vi "lab15_3-21_main.vi"() -> ()   [LabVIEW 2012]
uses:
  <vilib>/DAQmx/write.llb/DAQmx Write (Digital U8 1Chan 1Samp).vi
  <vilib>/DAQmx/create/channels.llb/DAQmx Create Channel (DO-Digital Output).vi
  <vilib>/DAQmx/miscellaneous.llb/DAQmx Fill In Error Info.vi
panel:
  out "out":u8 format="%08b"
  in  "Half-stepping":bool
  in  "Digital Port":tag
  in  "Number of steps\n(0 for run mode)":i32(knob) min=0 max=1000 scale=0.0..50.0
  in  "Stop Movement":bool
  in  "Move Right":bool
  in  "Move Left":bool
  in  "Terminate Program":bool
  in  "Speed":u8(knob)=1 max=7 step=1 scale=0.0..7.0
  # "Channel Configuration"
  # "Motor Operation"
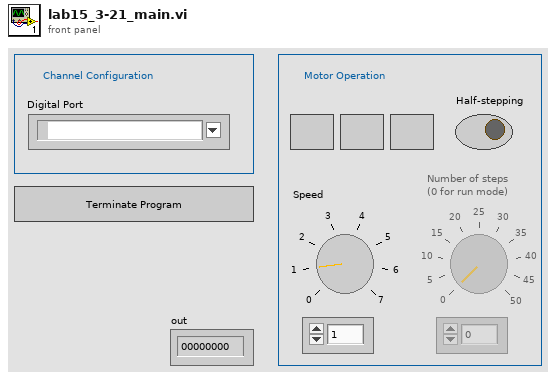
[diagram p1: front panel]
types:
  T1 = enum8{"Enabled", "Disabled", "Disabled and Grayed Out"}
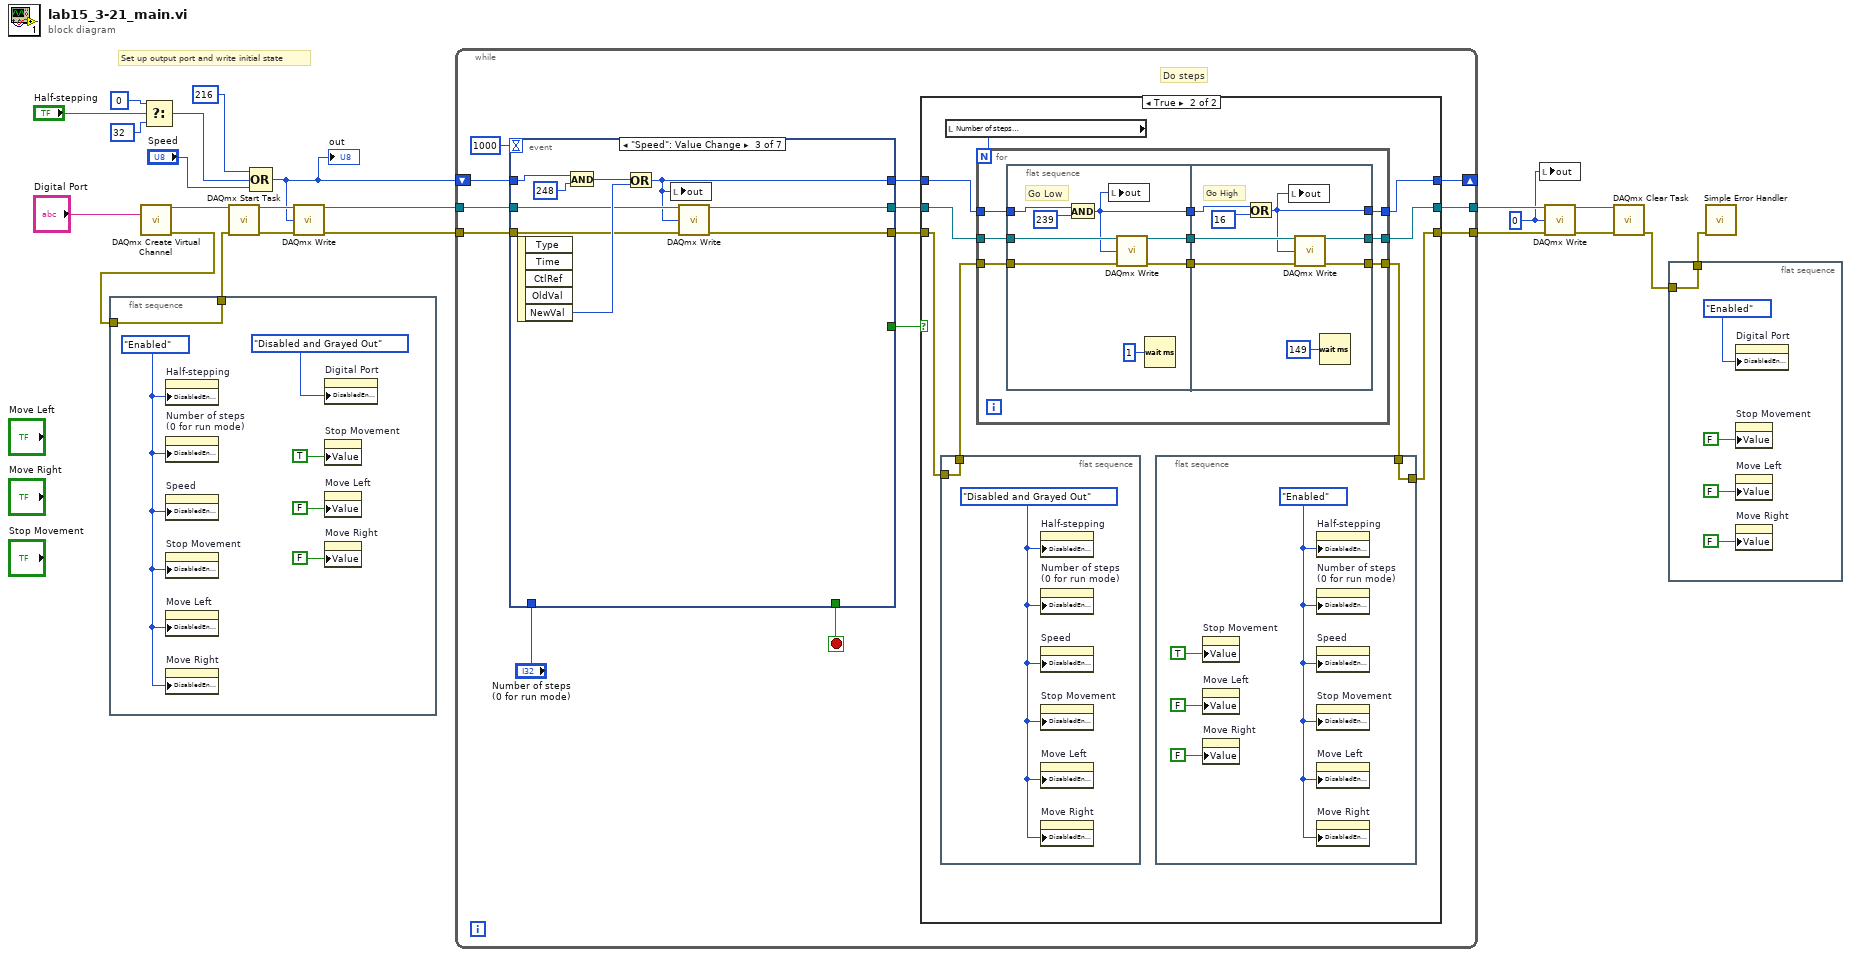
[diagram p0: block diagram]
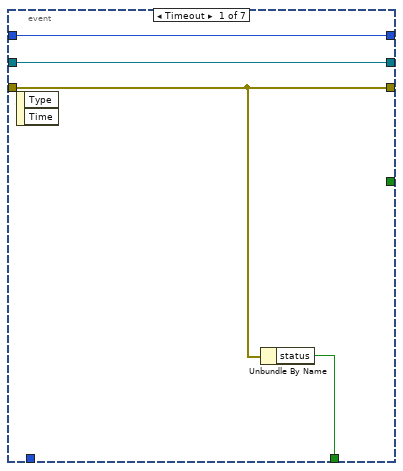
[diagram p3: hidden frame]
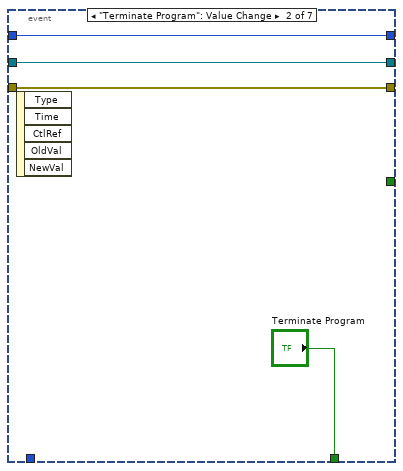
[diagram p4: hidden frame]
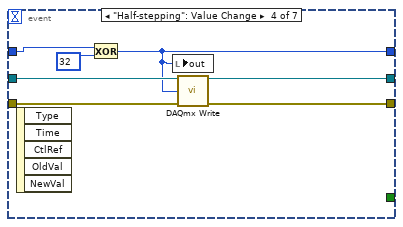
[diagram p5: hidden frame]
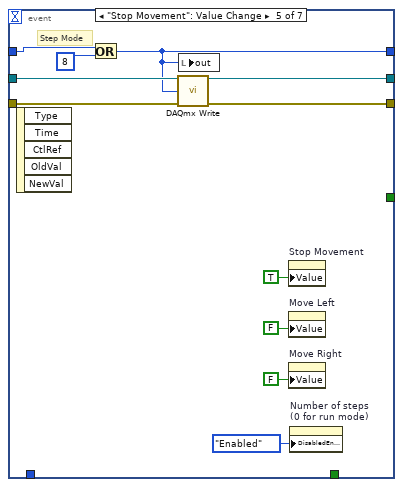
[diagram p6: hidden frame]
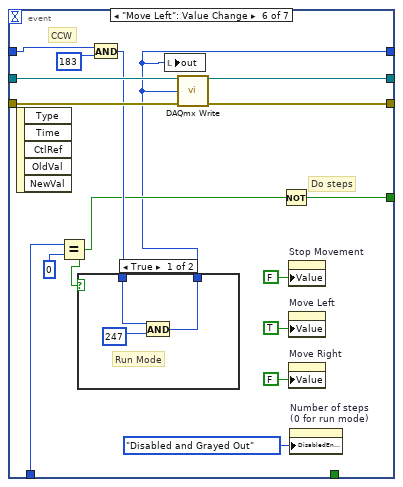
[diagram p7: hidden frame]
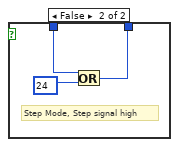
[diagram p8: hidden frame]
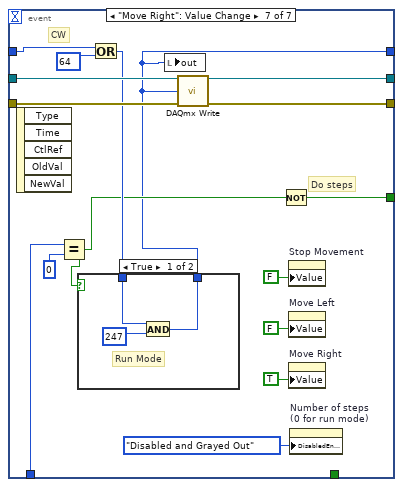
[diagram p9: hidden frame]
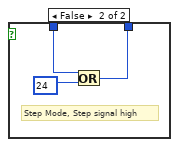
[diagram p10: hidden frame]
diagram:
  w2 = u8 0 ("data")
  # "Set up output port and write initial state"
  n1 = flat-sequence {
    tunnel: w8 -> [w28]
    tunnel: [w28] -> w7
    frame #0 {
      w27 = T1."Enabled" ("Disabled")
      n2 = property on="Half-stepping" class="Bool (strict)"("DisabledEnum"=w27) -> ()  [unwired: 2 in, 2 out]
      n3 = property on="Number of steps\n(0 for run mode)" class="Knob (strict)"("DisabledEnum"=w27) -> ()  [unwired: 2 in, 2 out]
      n4 = property on="Speed" class="Knob (strict)"("DisabledEnum"=w27) -> ()  [unwired: 2 in, 2 out]
      n5 = property on="Stop Movement" class="Bool (strict)"("DisabledEnum"=w27) -> ()  [unwired: 2 in, 2 out]
      n6 = property on="Move Left" class="Bool (strict)"("DisabledEnum"=w27) -> ()  [unwired: 2 in, 2 out]
      n7 = property on="Move Right" class="Bool (strict)"("DisabledEnum"=w27) -> ()  [unwired: 2 in, 2 out]
      n8 = property on="Digital Port" class="DAQmxName"("DisabledEnum"=T1."Disabled and Grayed Out" ("Disabled")) -> ()  [unwired: 2 in, 2 out]
      n9 = property on="Stop Movement" class="Bool (strict)"("Value"=TRUE ("Stop Movement")) -> ()  [unwired: 2 in, 2 out]
      n10 = property on="Move Left" class="Bool (strict)"("Value"=FALSE ("Move Left")) -> ()  [unwired: 2 in, 2 out]
      n11 = property on="Move Right" class="Bool (strict)"("Value"=FALSE ("Move Right")) -> ()  [unwired: 2 in, 2 out]
    }
  }
  n12 = call-poly <vilib>:"DAQmx Create Virtual Channel.vi"("lines"="Digital Port") -> ("task out"=w21:refnum<k21>, "error out"=w8:errorcluster)  [unwired: 13 in]
  n13 = Select(t=u8 0, s="Half-stepping", f=u8 32) -> (s? t:f=w9:u8)
  n14 = call <vilib>:"DAQmx Start Task.vi"("task/channels in"=w21, "error in"=w7) -> ("task out"=w18:refnum<k21>, "error out"=w17:errorcluster)  [unwired: 12 in]
  n15 = Compound Arithmetic op=OR(u8 216, w9, "Speed") -> (w1:u8)
  "out" <- w1
  n16 = call-poly <vilib>:"DAQmx Write.vi"("task/channels in"=w18, "data"=w1, "error in"=w17) -> ("task out"=w16:refnum<k21>, "error out"=w15:errorcluster)  [unwired: 10 in, 1 out]
  n17 = while {
    tunnel: w16 -> [w41]
    tunnel: w15 -> [w40]
    shift-right: [w34] -> _
    shift-left: w1 -> [w39]
    tunnel: [w32] -> w6
    tunnel: [w31] -> w5
    stop <- w38 stop-if-true
    # "Do steps"
    n18 = event shown="[2] \"Speed\": Value Change" {
      selector: _ -> [_ _ _ _ _ _ _]
      dyn-events: _ -> [_ _ _ _ _ _ _]
      timeout: 1000 -> [_ _ _ _ _ _ _]
      tunnel: w41 -> [w89 w91 w101 w109 w120 w136 w158]
      tunnel: w40 -> [w87 w90 w100 w108 w119 w135 w157]
      tunnel: [w89 w91 w98 w106 w117 w133 w155] -> w36
      tunnel: w39 -> [w88 w92 w95 w105 w116 w132 w154]
      tunnel: [w88 w92 w97 w103 w111 w122 w144] -> w37
      tunnel: [w86 "Terminate Program" _ _ _ _ _] -> w38
      tunnel: [w87 w90 w99 w107 w118 w134 w156] -> w35
      tunnel: [_ _ _ _ _ w124 w146] -> w33
      tunnel: "Number of steps\n(0 for run mode)" -> [_ _ _ _ _ w123 w145]
      event Timeout {
        n19 = event-data() -> ()  [unwired: 1 in, 2 out]
        n20 = Unbundle By Name(w87) -> ("status"=w86:bool)
      }
      event "Terminate Program": Value Change {
        n21 = event-data() -> ()  [unwired: 1 in, 5 out]
      }
      event "Speed": Value Change {
        n22 = event-data() -> ("NewVal"=w102:u8)  [unwired: 1 in, 4 out]
        n23 = And(x=w95, y=u8 248) -> (x .and. y?=w94:u8)
        n24 = Or(x=w94, y=w102) -> (x .or. y?=w97:u8)
        n25 = local write "out"(w97) -> ()
        n26 = call-poly <vilib>:"DAQmx Write.vi"("task/channels in"=w101, "data"=w97, "error in"=w100) -> ("task out"=w98:refnum<k21>, "error out"=w99:errorcluster)  [unwired: 10 in, 1 out]
      }
      event "Half-stepping": Value Change {
        n27 = event-data() -> ()  [unwired: 1 in, 5 out]
        n28 = Exclusive Or(1:u8 32, 2:w105) -> (0:w103:u8)
        n29 = local write "out"(w103) -> ()
        n30 = call-poly <vilib>:"DAQmx Write.vi"("task/channels in"=w109, "data"=w103, "error in"=w108) -> ("task out"=w106:refnum<k21>, "error out"=w107:errorcluster)  [unwired: 10 in, 1 out]
      }
      event "Stop Movement": Value Change {
        # "Step Mode"
        n31 = event-data() -> ()  [unwired: 1 in, 5 out]
        n32 = Or(x=w116, y=u8 8) -> (x .or. y?=w111:u8)
        n33 = call-poly <vilib>:"DAQmx Write.vi"("task/channels in"=w120, "data"=w111, "error in"=w119) -> ("task out"=w117:refnum<k21>, "error out"=w118:errorcluster)  [unwired: 10 in, 1 out]
        n34 = local write "out"(w111) -> ()
        n35 = property on="Stop Movement" class="Bool (strict)"("Value"=TRUE ("Stop Movement")) -> ()  [unwired: 2 in, 2 out]
        n36 = property on="Move Left" class="Bool (strict)"("Value"=FALSE ("Move Left")) -> ()  [unwired: 2 in, 2 out]
        n37 = property on="Move Right" class="Bool (strict)"("Value"=FALSE ("Move Left")) -> ()  [unwired: 2 in, 2 out]
        n38 = property on="Number of steps\n(0 for run mode)" class="Knob (strict)"("DisabledEnum"=T1."Enabled" ("Disabled")) -> ()  [unwired: 2 in, 2 out]
      }
      event "Move Left": Value Change {
        # "Do steps"
        # "CCW"
        n39 = event-data() -> ()  [unwired: 1 in, 5 out]
        n40 = Equal?(x=w123, y=0) -> (x = y?=w125:bool)
        n41 = And(x=w132, y=u8 183) -> (x .and. y?=w126:u8)
        n42 = case shown="True" w125 {
          tunnel: w126 -> [w139 w142]
          tunnel: [w137 w140] -> w122
          frame True {
            # "Run Mode"
            n43 = And(x=w139, y=u8 247) -> (x .and. y?=w137:u8)
          }
          frame False {
            # "Step Mode, Step signal high"
            n44 = Or(x=w142, y=u8 24) -> (x .or. y?=w140:u8)
          }
        }
        n45 = local write "out"(w122) -> ()
        n46 = call-poly <vilib>:"DAQmx Write.vi"("task/channels in"=w136, "data"=w122, "error in"=w135) -> ("task out"=w133:refnum<k21>, "error out"=w134:errorcluster)  [unwired: 10 in, 1 out]
        n47 = Not(x=w125) -> (.not. x?=w124:bool)
        n48 = property on="Stop Movement" class="Bool (strict)"("Value"=FALSE ("Stop Movement")) -> ()  [unwired: 2 in, 2 out]
        n49 = property on="Move Left" class="Bool (strict)"("Value"=TRUE ("Move Left")) -> ()  [unwired: 2 in, 2 out]
        n50 = property on="Move Right" class="Bool (strict)"("Value"=FALSE ("Move Left")) -> ()  [unwired: 2 in, 2 out]
        n51 = property on="Number of steps\n(0 for run mode)" class="Knob (strict)"("DisabledEnum"=T1."Disabled and Grayed Out" ("Disabled")) -> ()  [unwired: 2 in, 2 out]
      }
      event "Move Right": Value Change {
        # "Do steps"
        # "CW"
        n52 = event-data() -> ()  [unwired: 1 in, 5 out]
        n53 = Equal?(x=w145, y=0) -> (x = y?=w147:bool)
        n54 = Or(x=w154, y=u8 64) -> (x .or. y?=w148:u8)
        n55 = case shown="True" w147 {
          tunnel: w148 -> [w161 w164]
          tunnel: [w159 w162] -> w144
          frame True {
            # "Run Mode"
            n56 = And(x=w161, y=u8 247) -> (x .and. y?=w159:u8)
          }
          frame False {
            # "Step Mode, Step signal high"
            n57 = Or(x=w164, y=u8 24) -> (x .or. y?=w162:u8)
          }
        }
        n58 = local write "out"(w144) -> ()
        n59 = call-poly <vilib>:"DAQmx Write.vi"("task/channels in"=w158, "data"=w144, "error in"=w157) -> ("task out"=w155:refnum<k21>, "error out"=w156:errorcluster)  [unwired: 10 in, 1 out]
        n60 = Not(x=w147) -> (.not. x?=w146:bool)
        n61 = property on="Stop Movement" class="Bool (strict)"("Value"=FALSE ("Stop Movement")) -> ()  [unwired: 2 in, 2 out]
        n62 = property on="Move Left" class="Bool (strict)"("Value"=FALSE ("Move Left")) -> ()  [unwired: 2 in, 2 out]
        n63 = property on="Move Right" class="Bool (strict)"("Value"=TRUE ("Move Left")) -> ()  [unwired: 2 in, 2 out]
        n64 = property on="Number of steps\n(0 for run mode)" class="Knob (strict)"("DisabledEnum"=T1."Disabled and Grayed Out" ("Disabled")) -> ()  [unwired: 2 in, 2 out]
      }
    }
    n65 = case shown="True" w33 {
      tunnel: w37 -> [w44 w52]
      tunnel: w36 -> [w43 w51]
      tunnel: w35 -> [w42 w48]
      tunnel: [w44 w50] -> w34
      tunnel: [w43 w49] -> w32
      tunnel: [w42 w45] -> w31
      frame False {
      }
      frame True {
        n66 = flat-sequence {
          tunnel: w48 -> [w60]
          tunnel: [w60] -> w47
          frame #0 {
            w59 = T1."Disabled and Grayed Out" ("Disabled")
            n67 = property on="Half-stepping" class="Bool (strict)"("DisabledEnum"=w59) -> ()  [unwired: 2 in, 2 out]
            n68 = property on="Number of steps\n(0 for run mode)" class="Knob (strict)"("DisabledEnum"=w59) -> ()  [unwired: 2 in, 2 out]
            n69 = property on="Speed" class="Knob (strict)"("DisabledEnum"=w59) -> ()  [unwired: 2 in, 2 out]
            n70 = property on="Stop Movement" class="Bool (strict)"("DisabledEnum"=w59) -> ()  [unwired: 2 in, 2 out]
            n71 = property on="Move Left" class="Bool (strict)"("DisabledEnum"=w59) -> ()  [unwired: 2 in, 2 out]
            n72 = property on="Move Right" class="Bool (strict)"("DisabledEnum"=w59) -> ()  [unwired: 2 in, 2 out]
          }
        }
        n73 = local read "Number of steps\n(0 for run mode)"() -> (w53:i32)
        n74 = for {
          N: w53 -> [_]
          tunnel: w52 -> [w69]
          tunnel: w51 -> [w68]
          tunnel: w47 -> [w67]
          tunnel: [w63] -> w50
          tunnel: [w62] -> w49
          tunnel: [w61] -> w46
          n75 = flat-sequence {
            tunnel: w69 -> [w74]
            tunnel: w68 -> [w77]
            tunnel: w67 -> [w76]
            tunnel: [w70] -> w66
            tunnel: [w73] -> w65
            tunnel: [w72] -> w64
            tunnel: w66 -> [w84]
            tunnel: w65 -> [w83]
            tunnel: w64 -> [w82]
            tunnel: [w81] -> w62
            tunnel: [w80] -> w61
            tunnel: [w78] -> w63
            frame #0 {
              # "Go Low"
              n76 = And(x=w74, y=u8 239) -> (x .and. y?=w70:u8)
              n77 = local write "out"(w70) -> ()
              n78 = call-poly <vilib>:"DAQmx Write.vi"("task/channels in"=w77, "data"=w70, "error in"=w76) -> ("task out"=w73:refnum<k21>, "error out"=w72:errorcluster)  [unwired: 10 in, 1 out]
              n79 = Wait (ms)(milliseconds to wait=u32 1) -> ()  [unwired: 1 out]
            }
            frame #1 {
              # "Go High"
              n80 = Or(x=w84, y=u8 16) -> (x .or. y?=w78:u8)
              n81 = local write "out"(w78) -> ()
              n82 = call-poly <vilib>:"DAQmx Write.vi"("task/channels in"=w83, "data"=w78, "error in"=w82) -> ("task out"=w81:refnum<k21>, "error out"=w80:errorcluster)  [unwired: 10 in, 1 out]
              n83 = Wait (ms)(milliseconds to wait=u32 149) -> ()  [unwired: 1 out]
            }
          }
        }
        n84 = flat-sequence {
          tunnel: w46 -> [w57]
          tunnel: [w57] -> w45
          frame #0 {
            w58 = T1."Enabled" ("Disabled")
            n85 = property on="Stop Movement" class="Bool (strict)"("Value"=TRUE ("Stop Movement")) -> ()  [unwired: 2 in, 2 out]
            n86 = property on="Move Left" class="Bool (strict)"("Value"=FALSE ("Move Left")) -> ()  [unwired: 2 in, 2 out]
            n87 = property on="Move Right" class="Bool (strict)"("Value"=FALSE ("Move Right")) -> ()  [unwired: 2 in, 2 out]
            n88 = property on="Half-stepping" class="Bool (strict)"("DisabledEnum"=w58) -> ()  [unwired: 2 in, 2 out]
            n89 = property on="Number of steps\n(0 for run mode)" class="Knob (strict)"("DisabledEnum"=w58) -> ()  [unwired: 2 in, 2 out]
            n90 = property on="Speed" class="Knob (strict)"("DisabledEnum"=w58) -> ()  [unwired: 2 in, 2 out]
            n91 = property on="Stop Movement" class="Bool (strict)"("DisabledEnum"=w58) -> ()  [unwired: 2 in, 2 out]
            n92 = property on="Move Left" class="Bool (strict)"("DisabledEnum"=w58) -> ()  [unwired: 2 in, 2 out]
            n93 = property on="Move Right" class="Bool (strict)"("DisabledEnum"=w58) -> ()  [unwired: 2 in, 2 out]
          }
        }
      }
    }
  }
  n94 = local write "out"(w2) -> ()
  n95 = call-poly <vilib>:"DAQmx Write.vi"("task/channels in"=w6, "data"=w2, "error in"=w5) -> ("task out"=w20:refnum<k21>, "error out"=w19:errorcluster)  [unwired: 10 in, 1 out]
  n96 = call <vilib>:"DAQmx Clear Task.vi"("task in"=w20, "error in"=w19) -> ("error out"=w4:errorcluster)  [unwired: 13 in]
  n97 = flat-sequence {
    tunnel: w4 -> [w169]
    tunnel: [w169] -> w3
    frame #0 {
      n98 = property on="Digital Port" class="DAQmxName"("DisabledEnum"=T1."Enabled" ("Disabled")) -> ()  [unwired: 2 in, 2 out]
      n99 = property on="Stop Movement" class="Bool (strict)"("Value"=FALSE ("Stop Movement")) -> ()  [unwired: 2 in, 2 out]
      n100 = property on="Move Left" class="Bool (strict)"("Value"=FALSE ("Move Left")) -> ()  [unwired: 2 in, 2 out]
      n101 = property on="Move Right" class="Bool (strict)"("Value"=FALSE ("Move Right")) -> ()  [unwired: 2 in, 2 out]
    }
  }
  n102 = call <vilib>:"Simple Error Handler.vi"("error in (no error)"=w3) -> ()  [unwired: 4 in, 5 out]
